vi "Timer Create.vi"(8 "error in (no error)":errorcluster) -> (0 "error out":errorcluster, 3 "Timer reference out":refnum<data-value>)   [LabVIEW 2018]
doc: "This VI is part of a Timer class that is implemented with the DVR. It creates the Timer.\n\nAAL 9/09"
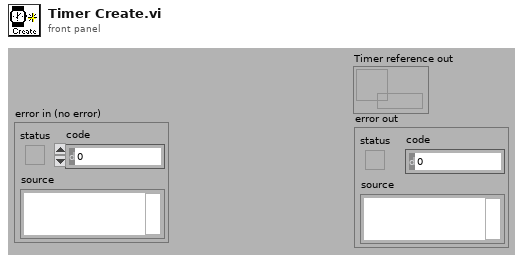
[diagram p1: front panel]
types:
  T1 = cluster{"Start Time":i32, "Elapsed Time":i32, "Running?":bool}
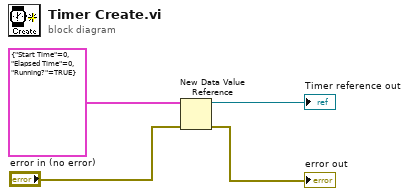
[diagram p0: block diagram]
diagram:
  n1 = New Data Value Reference(data value=T1 {"Start Time"=0, "Elapsed Time"=0, "Running?"=TRUE}, error in="error in (no error)") -> (data value reference=→"Timer reference out":refnum<data-value>, error out=→"error out":errorcluster)
